vi "OpenFPGA.vi"(10 "FPGA bit file path":string, 11 "Resource name":string="PXI-7821R") -> (0 "Error code":i32, 3 "Reference ID":u64)   [LabVIEW 2023]
doc: "Opens FPGA reference using bitfile and RIO device. \nNote: Bitfile should be built for the exact type of RIO device."
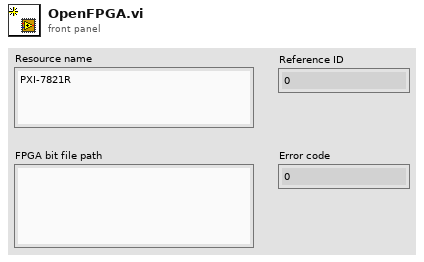
[diagram p1: front panel]
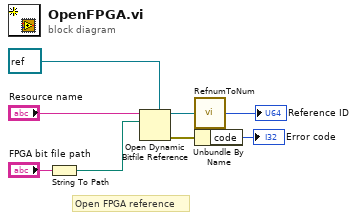
[diagram p0: block diagram]
diagram:
  # "Open FPGA reference"
  n1 = String To Path(string="FPGA bit file path") -> (path=w1:path)
  n2 = Open Dynamic Bitfile Reference(0:"Resource name", 1:w1, 4:refnum<k20> refnum ("FPGA VI Reference Out")) -> (5:w3:refnum<k20>, 8:w5:errorcluster)  [unwired: 2 in]
  n3 = call "RefnumToNum.vi"("Refnum in"=w3) -> ("Reference ID"=→"Reference ID":u64)
  n4 = Unbundle By Name(w5) -> ("code"=→"Error code":i32)
